vi "EditAttribute__slk_msxml.vi"(0 "document in":refnum<class "msxml document.lvclass">, 5 "node in":refnum<class "msxml node.lvclass">, 11 "error in (no error)":errorcluster, 12 "attributes":T1) -> (4 "document out":refnum<class "msxml document.lvclass">, 6 "node out":refnum<class "msxml node.lvclass">, 15 "error out":errorcluster)   [LabVIEW 2020, in "MSXML.lvlib" / "msxml node.lvclass"]
doc: "Modifies node attributes value by specified node."
uses:
  msxml node.lvclass
  MSXML Document/msxml document.lvclass
  Type Definition/Attributes__slk_msxml.ctl
  Type Definition/Attribute__slk_msxml.ctl
  msxml node.lvclass/msxml node.ctl
  MSXML.lvlib
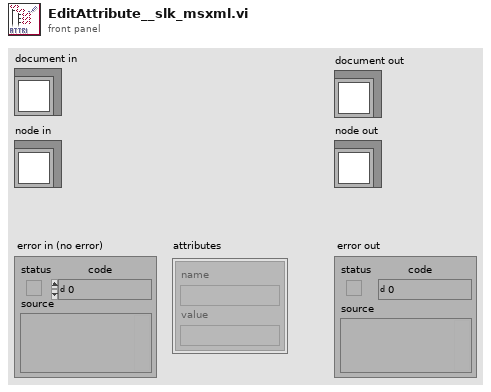
[diagram p1: front panel]
types:
  T1 = typedef "MSXML.lvlib/Attributes__slk_msxml.ctl" = T2[]
  T2 = typedef "MSXML.lvlib/Attribute__slk_msxml.ctl" = cluster{"name":string, "value":string}
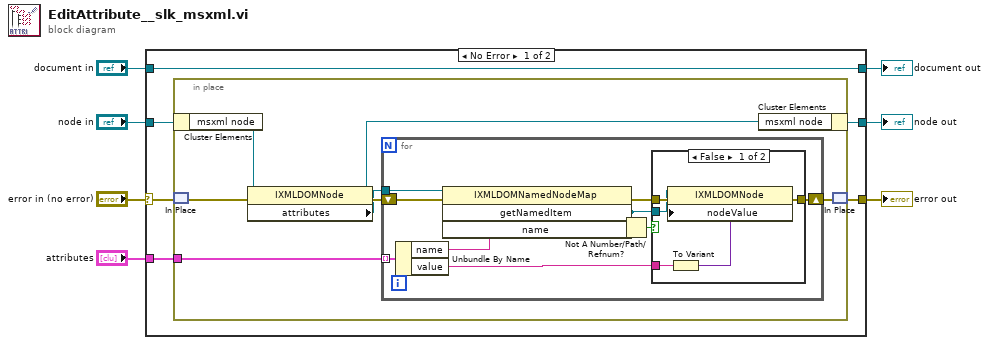
[diagram p0: block diagram]
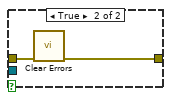
[diagram p2: hidden frame]
diagram:
  n1 = case shown="No Error" "error in (no error)" {
    selector: "error in (no error)" -> [w13 w39]
    tunnel: "document in" -> [w10 w38]
    tunnel: [w12 w39] -> w5
    tunnel: "node in" -> [w11 w37]
    tunnel: [w10 w38] -> w3
    tunnel: [w9 w37] -> w2
    tunnel: "attributes" -> [w8 _]
    frame No Error {
      n2 = in-place {
        in-place-border: w8 -> [w16]
        n3 = in-place-cluster #1(w11) -> ("msxml node"=w18:refnum<k7>)
        n4 = in-place-match #2(w13) -> (w17:errorcluster)
        n5 = property class="IXMLDOMNode"(reference=w18, error in=w17) -> (reference out=w14:refnum<k7>, error out=w20:errorcluster, "attributes"=w19:refnum<k7>)
        n6 = for {
          tunnel: w19 -> [w28]
          shift-right: [w22] -> w15
          shift-left: w20 -> [w29]
          tunnel: w16 -> [w27] mode=indexing
          n7 = Unbundle By Name(w27) -> ("name"=w26:string, "value"=w21:string)
          n8 = invoke class="IXMLDOMNamedNodeMap" method="getNamedItem"(reference=w28, error in=w29, "name"=w26) -> (error out=w24:errorcluster, "getNamedItem"=w23:refnum<k7>)  [unwired: 1 in, 2 out]
          n9 = Not A Number/Path/Refnum?(number/path/refnum=w23) -> (NaN/Path/Refnum?=w25:bool)
          n10 = case shown="False" w25 {
            tunnel: w24 -> [w34 w36]
            tunnel: w23 -> [w32 _]
            tunnel: [w33 w35] -> w22
            tunnel: w21 -> [w31 _]
            frame False {
              n11 = To Variant(anything=w31) -> (Variant=w30:variant)
              n12 = property class="IXMLDOMNode"(reference=w32, error in=w34, "nodeValue"=w30) -> (error out=w33:errorcluster)  [unwired: 1 out]
            }
            frame True {
              n13 = call <vilib>:"Clear Errors.vi"("error in (no error)"=w36) -> ("error out"=w35:errorcluster)  [unwired: 5 in, 1 out]
            }
          }
        }
        n14 = in-place-cluster #1("msxml node"=w14) -> (w9:refnum<class "msxml node.lvclass">)
        n15 = in-place-match #2(w15) -> (w12:errorcluster)
      }
    }
    frame Error {
    }
  }
  "node out" <- w2
  "document out" <- w3
  "error out" <- w5
